vi "Ini_Ovens.vi"(8 "error in (no error)":errorcluster) -> (0 "error out":errorcluster, 3 "Овны":refnum<class "Modbus Master.lvclass">[](array[class]))   [LabVIEW 2018]
uses:
  <vilib>/NI/Modbus Library/API/Master/Modbus Master.lvclass
  <vilib>/NI/Modbus Library/API/Wrapper/Create TCP Master.vi
  <vilib>/NI/Modbus Library/API/Wrapper/API Main.lvlib
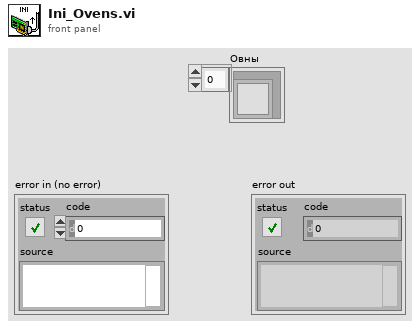
[diagram p1: front panel]
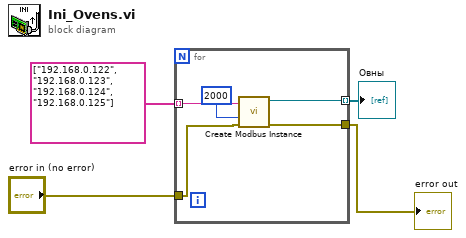
[diagram p0: block diagram]
diagram:
  n1 = for {
    tunnel: string[] ["192.168.0.122", "192.168.0.123", "192.168.0.124", "192.168.0.125"] -> [w9] mode=indexing
    tunnel: [w8] -> w1 mode=indexing
    tunnel: [w7] -> w3
    tunnel: "error in (no error)" -> [w6]
    n2 = call-poly <vilib>:"Create Modbus Instance.vi"("error in"=w6, "connect timeout ms"=2000, "address"=w9) -> ("error out"=w7:errorcluster, "TCP master instance"=w8:refnum<class "Modbus Master.lvclass">)  [unwired: 7 in]
  }
  "error out" <- w3
  "Овны" <- w1
